vi "MotorPositionController PositionChangeEvent Example.vi"() -> ()   [LabVIEW 2012, in "Phidget Motor Position Controller.lvlib"]
uses:
  <instrlib>/Phidgets/Phidget Motor Position Controller/Phidget Motor Position Controller.lvlib
  <instrlib>/Phidgets/Phidget Motor Position Controller/Public/MotorPositionControllerStart.vi
  <instrlib>/Phidgets/Phidget Motor Position Controller/Public/MotorPositionControllerClose.vi
  <instrlib>/Phidgets/Phidget Common/Phidget Common.lvlib
panel:
  in  "MotorPosCtrl Init Data":T1={"Rescale Factor"=1.0, "Velocity Limit"=20000.0, "Acceleration"=10000.0, "Kp"=2000.0, "Ki"=5.0, "Kd"=25000.0, "DeadBand"=0.0}
  in  "Target Position":dbl=10000.0 caption="Position"
  in  "Engaged":bool=TRUE
  out "Position Return":dbl caption="Duty Cycle Return"
  in  "stop":bool
  out "Serial Number Return":i32
  in  "Device Info":T2={"Serial Number"=-1, "Channel"=0, "Port"=0}
  out "error out":errorcluster
  # "Be sure to use this stop button to stop the program.\nIf you use the \"Abort Execution\" button, you will\nneed to use PhidgetResetLibrary.vi or restart Labview \nin order for any Phidgets to work."
  # "The default Velocity Limit and Acceleration settings seen here are not compatible with the DCC1100 BLDC Motor controller. They may both be set  to 200 (or some other compatible value) for \nthe device to work."
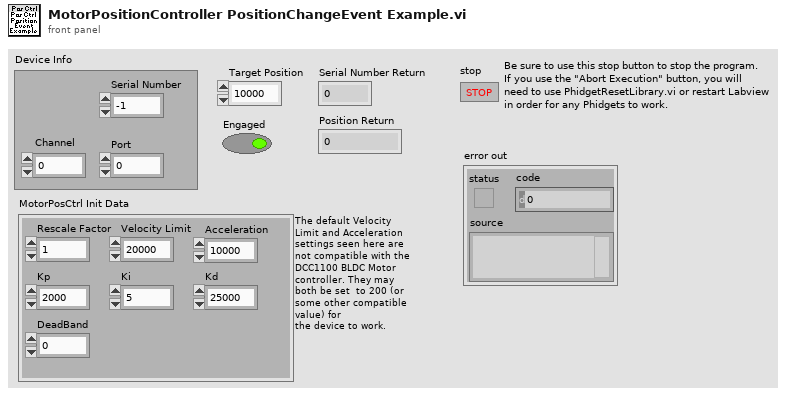
[diagram p1: front panel]
types:
  T1 = cluster{"Rescale Factor":dbl, "Velocity Limit":dbl, "Acceleration":dbl, "Kp":dbl, "Ki":dbl, "Kd":dbl, "DeadBand":dbl}
  T2 = cluster{"Serial Number":i32, "Channel":i32, "Port":i32}
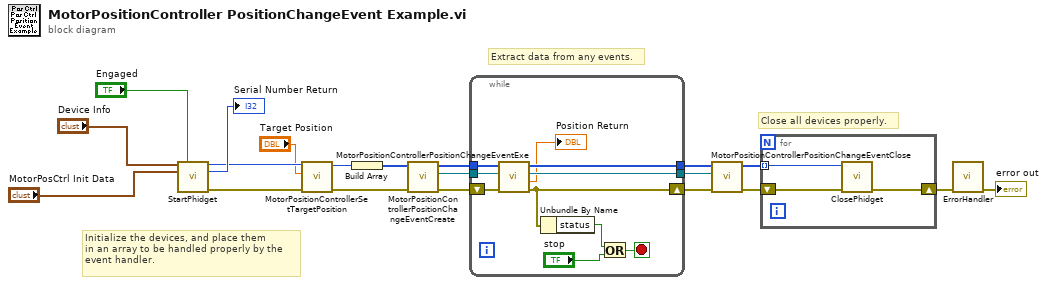
[diagram p0: block diagram]
diagram:
  # "Close all devices properly."
  # "Extract data from any events."
  # "Initialize the devices, and place them\nin an array to be handled properly by the\nevent handler."
  n1 = call-poly <instrlib>:"StartPhidget.vi"("Device Info"="Device Info", "Engaged"="Engaged", "MotorPosCtrl Init Data"="MotorPosCtrl Init Data") -> ("Phidget ID"=w6:u64, "Serial Number Return"=→"Serial Number Return":i32, "error out"=w5:errorcluster)  [unwired: 9 in, 1 out]
  n2 = call <instrlib>:"MotorPositionControllerSetTargetPosition.vi"("error in (no error)"=w5, "Position"="Target Position", "Device In"=w6) -> ("error out"=w2:errorcluster, "Device Out"=w3:u64)  [unwired: 6 in]
  n3 = Build Array(w3) -> (w20:u64[])
  n4 = call <instrlib>:"MotorPositionControllerPositionChangeEventCreate.vi"("error in (no error)"=w2, "Devices In"=w20) -> ("error out"=w13:errorcluster, "Event Registration Refnum"=w18:refnum<event-registration>, "Devices Out"=w19:u64[])  [unwired: 7 in]
  n5 = while {
    tunnel: w19 -> [w30]
    tunnel: w18 -> [w27]
    tunnel: [w22] -> w15
    shift-right: [w23] -> w14
    shift-left: w13 -> [w29]
    tunnel: [w28] -> w9
    stop <- w26 stop-if-true
    n6 = call <instrlib>:"MotorPositionControllerPositionChangeEventExe.vi"("error in (no error)"=w29, "Event Registration Refnum In"=w27, "Devices In"=w30) -> ("error out"=w23:errorcluster, "Position"=→"Position Return":dbl, "Event Registration Refnum"=w22:refnum<event-registration>, "Devices Out"=w28:u64[])  [unwired: 2 in, 3 out]
    n7 = Unbundle By Name(w23) -> ("status"=w24:bool)
    n8 = Or(x=w24, y="stop") -> (x .or. y?=w26:bool)
  }
  n9 = call <instrlib>:"MotorPositionControllerPositionChangeEventClose.vi"("error in (no error)"=w14, "Event Registration Refnum In"=w15, "Devices In"=w9) -> ("error out"=w11:errorcluster, "Devices Out"=w10:u64[])  [unwired: 7 in]
  n10 = for {
    tunnel: w10 -> [w32] mode=indexing
    shift-right: [w33] -> w17
    shift-left: w11 -> [w31]
    n11 = call-poly <instrlib>:"ClosePhidget.vi"("error in"=w31, "Device In"=w32) -> ("error out"=w33:errorcluster)  [unwired: 9 in]
  }
  n12 = call <instrlib>:"ErrorHandler.vi"("error in"=w17) -> ("error out"=→"error out":errorcluster)  [unwired: 9 in, 1 out]
